vi "Disconnection.vi"(8 "error in (no error)":errorcluster, 11 "SIMATIC_S7 in":refnum<class "SIMATIC_S7.lvclass">) -> (0 "error out":errorcluster, 3 "SIMATIC_S7 out":refnum<class "SIMATIC_S7.lvclass">)   [LabVIEW 2025, in "SIMATIC_S7.lvclass"]
uses:
  SIMATIC_S7.lvclass
  SIMATIC_S7.lvclass/SIMATIC_S7.ctl
  <vilib>/Hampel Software Engineering/S7NetCom/Source/S7NetCom.lvclass
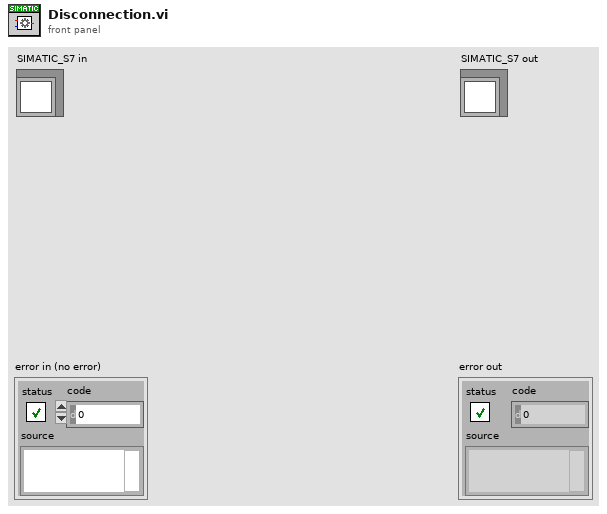
[diagram p1: front panel]
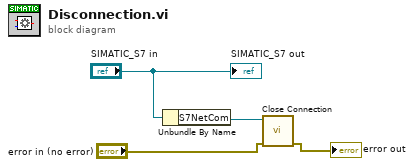
[diagram p0: block diagram]
diagram:
  n1 = Unbundle By Name("SIMATIC_S7 in") -> ("S7NetCom"=w3:refnum<class "S7NetCom.lvclass">)
  n2 = call <vilib>:"Close Connection.vi"("error in (no error)"="error in (no error)", "S7NetCom in"=w3) -> ("error out"=→"error out":errorcluster)  [unwired: 8 in, 1 out]
  "SIMATIC_S7 out" <- "SIMATIC_S7 in"
